vi "SP Convert 4.3 to 4.4.vi"(0 "S Parameter 4.3 Test Parameters":T2={"Stimulus"={"Use Instrument Settings"=FALSE, "Blank Frequencies"=FALSE, "Sweep Type"=enum."Linear", "Sweep"={"Fstart"=0.0, "Fstop"=0.0, "Units"=enum."Hz", "Points"=2}, "Power (dBm)"=999.0, "IFBW (Hz)"=-1.0, "Sweep Time (s)"=-1.0}, "Measurement"={"Auto Select"=FALSE, "Data Source"=enum."VNA", "Ports"=2, "Calibration"={"State"=FALSE, "String"=""}, "Parameters"=[]}, "De-Embed"={"De-Embed"=FALSE, "Adapters"=[]}, "Display"={"Lock Control"=FALSE, "Retain Settings"=FALSE, "Formatted Data"=FALSE, "Plot Orientation"=enum."Single", "Plot Controls"=[{"Trace Orientation"=enum."Overlay", "Frequency"={"Change Frequency"=FALSE, "Start"=500.0, "Stop"=1500.0, "Units"=enum."MHz"}, "Markers (MHz)"=[], "Traces"=[{"Trace On"=TRUE, "Measure"=0, "Format"=0, "Autoscale"=TRUE, "Reference"=0.0, "\nRefUnit"="dB/Div", "Position"=5.0, "Scale"=10.0, "ScaleUnit"="dB/Div", "LimitOn"=TRUE, "LimitFill"=FALSE, "Display Data"=0, "Show Markers"=FALSE, "SXX"=""}, {"Trace On"=TRUE, "Measure"=0, "Format"=0, "Autoscale"=TRUE, "Reference"=0.0, "\nRefUnit"="dB/Div", "Position"=5.0, "Scale"=10.0, "ScaleUnit"="dB/Div", "LimitOn"=TRUE, "LimitFill"=FALSE, "Display Data"=0, "Show Markers"=FALSE, "SXX"=""}]}, {"Trace Orientation"=enum."Overlay", "Frequency"={"Change Frequency"=FALSE, "Start"=500.0, "Stop"=1500.0, "Units"=enum."MHz"}, "Markers (MHz)"=[], "Traces"=[{"Trace On"=TRUE, "Measure"=0, "Format"=0, "Autoscale"=TRUE, "Reference"=0.0, "\nRefUnit"="dB/Div", "Position"=5.0, "Scale"=10.0, "ScaleUnit"="dB/Div", "LimitOn"=TRUE, "LimitFill"=FALSE, "Display Data"=0, "Show Markers"=FALSE, "SXX"=""}, {"Trace On"=TRUE, "Measure"=0, "Format"=0, "Autoscale"=TRUE, "Reference"=0.0, "\nRefUnit"="dB/Div", "Position"=5.0, "Scale"=10.0, "ScaleUnit"="dB/Div", "LimitOn"=TRUE, "LimitFill"=FALSE, "Display Data"=0, "Show Markers"=FALSE, "SXX"=""}]}, {"Trace Orientation"=enum."Overlay", "Frequency"={"Change Frequency"=FALSE, "Start"=500.0, "Stop"=1500.0, "Units"=enum."MHz"}, "Markers (MHz)"=[], "Traces"=[{"Trace On"=TRUE, "Measure"=0, "Format"=0, "Autoscale"=TRUE, "Reference"=0.0, "\nRefUnit"="dB/Div", "Position"=5.0, "Scale"=10.0, "ScaleUnit"="dB/Div", "LimitOn"=TRUE, "LimitFill"=FALSE, "Display Data"=0, "Show Markers"=FALSE, "SXX"=""}, {"Trace On"=TRUE, "Measure"=0, "Format"=0, "Autoscale"=TRUE, "Reference"=0.0, "\nRefUnit"="dB/Div", "Position"=5.0, "Scale"=10.0, "ScaleUnit"="dB/Div", "LimitOn"=TRUE, "LimitFill"=FALSE, "Display Data"=0, "Show Markers"=FALSE, "SXX"=""}]}, {"Trace Orientation"=enum."Overlay", "Frequency"={"Change Frequency"=FALSE, "Start"=500.0, "Stop"=1500.0, "Units"=enum."MHz"}, "Markers (MHz)"=[], "Traces"=[{"Trace On"=TRUE, "Measure"=0, "Format"=0, "Autoscale"=TRUE, "Reference"=0.0, "\nRefUnit"="dB/Div", "Position"=5.0, "Scale"=10.0, "ScaleUnit"="dB/Div", "LimitOn"=TRUE, "LimitFill"=FALSE, "Display Data"=0, "Show Markers"=FALSE, "SXX"=""}, {"Trace On"=TRUE, "Measure"=0, "Format"=0, "Autoscale"=TRUE, "Reference"=0.0, "\nRefUnit"="dB/Div", "Position"=5.0, "Scale"=10.0, "ScaleUnit"="dB/Div", "LimitOn"=TRUE, "LimitFill"=FALSE, "Display Data"=0, "Show Markers"=FALSE, "SXX"=""}]}]}, "Limits"=[]} {"Measurement"."Parameters"."Channel" min=0 max=32 step=1; "Stimulus"."Sweep Time (s)" format="%.3g"; "Display"."Plot Controls"."Traces"."Reference" format="%#.2g"; "Display"."Plot Controls"."Traces"."Display Data" items=["Data", "Memory", "Data/Memory"]; "Display"."Plot Controls"."Traces"."Format" items=["Log Mag", "Phase", "Delay", "Smith", "Polar", "Lin Mag", "SWR", "Loss", "Real", "Imaginary"]; "Display"."Plot Controls"."Traces"."Scale" min=0.001 step=1.0 format="%#.2g"; "Display"."Plot Controls"."Traces"."Position" min=0.0 max=10.0; "Display"."Plot Controls"."Frequency"."Stop" format="%.3g"; "Display"."Plot Controls"."Frequency"."Start" format="%.3g"}) -> (2 "S Parameter 4.4 - 4.5 Test Parameters":T1={"Stimulus"={"Use Instrument Settings"=FALSE, "Blank Frequencies"=FALSE, "Sweep Type"=enum."Linear", "Sweep"={"Fstart"=0.0, "Fstop"=0.0, "Units"=enum."Hz", "Points"=2}, "Power (dBm)"=999.0, "IFBW (Hz)"=-1.0, "Sweep Time (s)"=-1.0}, "Measurement"={"Auto Select"=TRUE, "Data Source"=enum."VNA", "Ports"=2, "Calibration"={"State"=FALSE, "String"=""}, "Parameters"=[]}, "De-Embed"={"De-Embed"=FALSE, "Adapters"=[]}, "Display"={"Lock Control"=FALSE, "Retain Settings"=TRUE, "Formatted Data"=FALSE, "Plot Orientation"=enum."Single", "Plot Controls"=[{"Trace Orientation"=enum."Overlay", "Frequency"={"Change Frequency"=FALSE, "Start"=500.0, "Stop"=1500.0, "Units"=enum."MHz"}, "Markers (MHz)"=[], "Traces"=[{"Trace On"=TRUE, "Measure"=0, "Format"=0, "Autoscale"=TRUE, "Reference"=0.0, "\nRefUnit"="dB/Div", "Position"=5.0, "Scale"=10.0, "ScaleUnit"="dB/Div", "LimitOn"=TRUE, "LimitFill"=FALSE, "Display Data"=0, "Show Markers"=FALSE, "SXX"=""}, {"Trace On"=TRUE, "Measure"=0, "Format"=0, "Autoscale"=TRUE, "Reference"=0.0, "\nRefUnit"="dB/Div", "Position"=5.0, "Scale"=10.0, "ScaleUnit"="dB/Div", "LimitOn"=TRUE, "LimitFill"=FALSE, "Display Data"=0, "Show Markers"=FALSE, "SXX"=""}]}, {"Trace Orientation"=enum."Overlay", "Frequency"={"Change Frequency"=FALSE, "Start"=500.0, "Stop"=1500.0, "Units"=enum."MHz"}, "Markers (MHz)"=[], "Traces"=[{"Trace On"=TRUE, "Measure"=0, "Format"=0, "Autoscale"=TRUE, "Reference"=0.0, "\nRefUnit"="dB/Div", "Position"=5.0, "Scale"=10.0, "ScaleUnit"="dB/Div", "LimitOn"=TRUE, "LimitFill"=FALSE, "Display Data"=0, "Show Markers"=FALSE, "SXX"=""}, {"Trace On"=TRUE, "Measure"=0, "Format"=0, "Autoscale"=TRUE, "Reference"=0.0, "\nRefUnit"="dB/Div", "Position"=5.0, "Scale"=10.0, "ScaleUnit"="dB/Div", "LimitOn"=TRUE, "LimitFill"=FALSE, "Display Data"=0, "Show Markers"=FALSE, "SXX"=""}]}, {"Trace Orientation"=enum."Overlay", "Frequency"={"Change Frequency"=FALSE, "Start"=500.0, "Stop"=1500.0, "Units"=enum."MHz"}, "Markers (MHz)"=[], "Traces"=[{"Trace On"=TRUE, "Measure"=0, "Format"=0, "Autoscale"=TRUE, "Reference"=0.0, "\nRefUnit"="dB/Div", "Position"=5.0, "Scale"=10.0, "ScaleUnit"="dB/Div", "LimitOn"=TRUE, "LimitFill"=FALSE, "Display Data"=0, "Show Markers"=FALSE, "SXX"=""}, {"Trace On"=TRUE, "Measure"=0, "Format"=0, "Autoscale"=TRUE, "Reference"=0.0, "\nRefUnit"="dB/Div", "Position"=5.0, "Scale"=10.0, "ScaleUnit"="dB/Div", "LimitOn"=TRUE, "LimitFill"=FALSE, "Display Data"=0, "Show Markers"=FALSE, "SXX"=""}]}, {"Trace Orientation"=enum."Overlay", "Frequency"={"Change Frequency"=FALSE, "Start"=500.0, "Stop"=1500.0, "Units"=enum."MHz"}, "Markers (MHz)"=[], "Traces"=[{"Trace On"=TRUE, "Measure"=0, "Format"=0, "Autoscale"=TRUE, "Reference"=0.0, "\nRefUnit"="dB/Div", "Position"=5.0, "Scale"=10.0, "ScaleUnit"="dB/Div", "LimitOn"=TRUE, "LimitFill"=FALSE, "Display Data"=0, "Show Markers"=FALSE, "SXX"=""}, {"Trace On"=TRUE, "Measure"=0, "Format"=0, "Autoscale"=TRUE, "Reference"=0.0, "\nRefUnit"="dB/Div", "Position"=5.0, "Scale"=10.0, "ScaleUnit"="dB/Div", "LimitOn"=TRUE, "LimitFill"=FALSE, "Display Data"=0, "Show Markers"=FALSE, "SXX"=""}]}]}, "Limits"=[]} {"Measurement"."Parameters"."Channel" min=0 max=32 step=1; "Measurement"."Parameters"."Parameter"."Stimulus Port" min=1 step=1; "Measurement"."Parameters"."Parameter"."Response Port" min=1 step=1; "Limits"."Parameter"."Stimulus Port" min=1 step=1; "Limits"."Parameter"."Response Port" min=1 step=1; "Stimulus"."Sweep Time (s)" format="%.3g"; "Display"."Plot Controls"."Traces"."Reference" format="%#.2g"; "Display"."Plot Controls"."Traces"."Display Data" items=["Data", "Memory", "Data/Memory"]; "Display"."Plot Controls"."Traces"."Format" items=["Log Mag", "Phase", "Expanded Phase", "Delay", "Smith", "Polar", "Lin Mag", "SWR", "Loss", "Real", "Imaginary"]; "Display"."Plot Controls"."Traces"."Scale" min=0.001 step=1.0 format="%#.2g"; "Display"."Plot Controls"."Traces"."Position" min=0.0 max=10.0; "Display"."Plot Controls"."Frequency"."Stop" format="%.3g"; "Display"."Plot Controls"."Frequency"."Start" format="%.3g"})   [LabVIEW 2011]
uses:
  TypeDefs/SP Test Parameters v4.3.ctl
  TypeDefs/SP Test Parameters v4.4-4.5.ctl
panel:
  # "Div"
  # "Div"
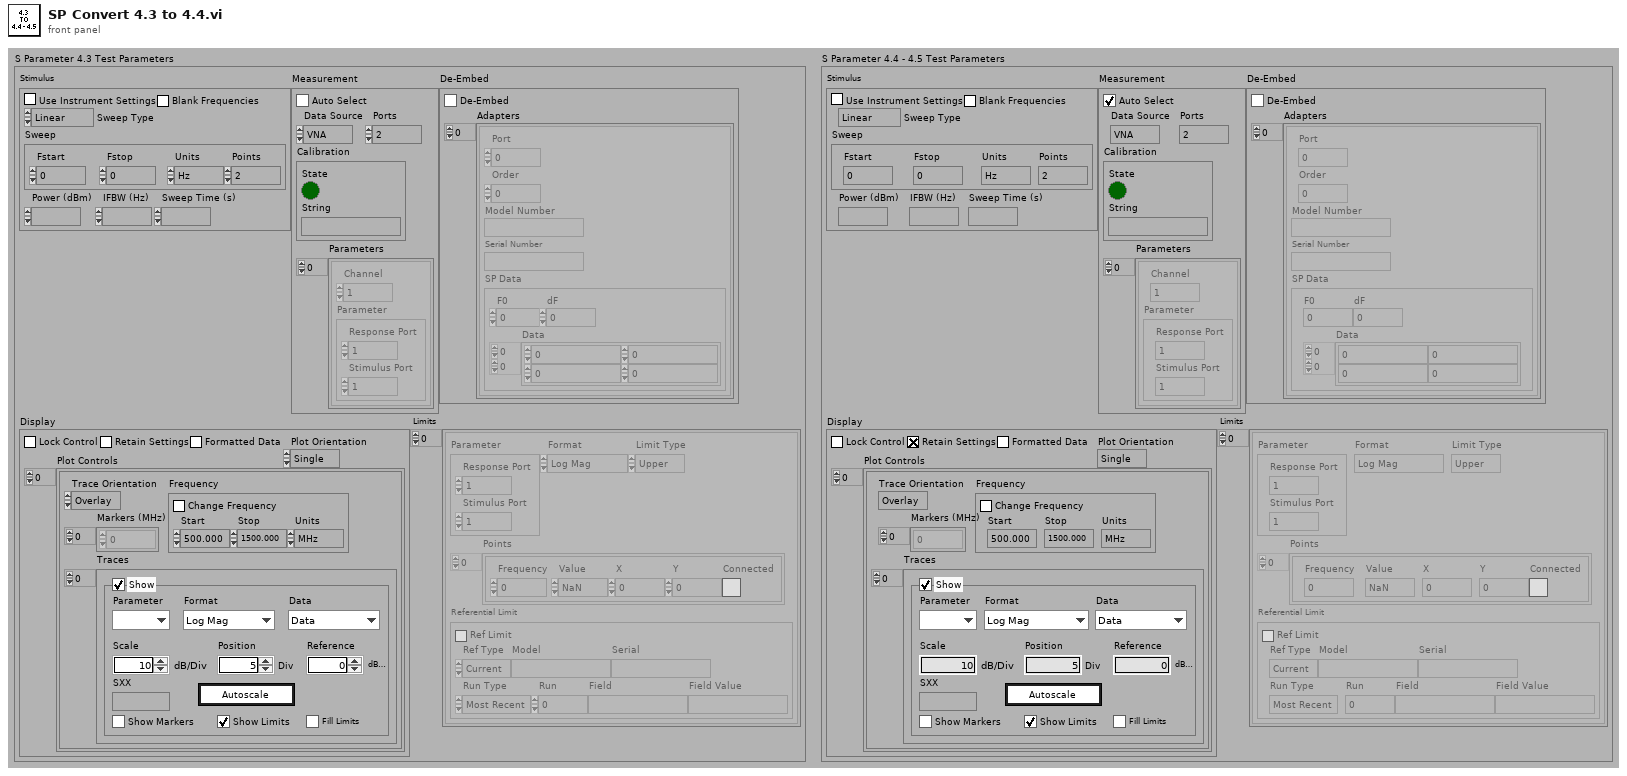
[diagram p1: front panel]
types:
  T1 = typedef "SP Test Parameters v4.4-4.5.ctl" = cluster{"Stimulus":cluster{"Use Instrument Settings":bool, "Blank Frequencies":bool, "Sweep Type":enum32{"Linear", "Logarithmic", "List", "Power", "CW"}, "Sweep":cluster{"Fstart":dbl, "Fstop":dbl, "Units":enum16{"Hz", "kHz", "MHz", "GHz", "Points"}, "Points":i32}, "Power (dBm)":dbl, "IFBW (Hz)":dbl, "Sweep Time (s)":dbl}, "Measurement":cluster{"Auto Select":bool, "Data Source":enum16{"VNA", "Data File"}, "Ports":i8, "Calibration":cluster{"State":bool, "String":string}, "Parameters":cluster{"Channel":i8, "Parameter":cluster{"Stimulus Port":i8, "Response Port":i8}}[]}, "De-Embed":cluster{"De-Embed":bool, "Adapters":cluster{"Port":i8, "Order":i8, "Model Number":string, "Serial Number":string, "SP Data":cluster{"F0":dbl, "dF":dbl, "Data":cdb[][]}}[]}, "Display":cluster{"Lock Control":bool, "Retain Settings":bool, "Formatted Data":bool, "Plot Orientation":enum32{"Single", "Dual", "Quad"}, "Plot Controls":cluster{"Trace Orientation":enum32{"Overlay", "Split"}, "Frequency":cluster{"Change Frequency":bool, "Start":dbl, "Stop":dbl, "Units":enum16{"Hz", "kHz", "MHz", "GHz", "Points"}}, "Markers (MHz)":dbl[], "Traces":cluster{"Trace On":bool, "Measure":i32, "Format":i32, "Autoscale":bool, "Reference":dbl, "\nRefUnit":string, "Position":dbl, "Scale":dbl, "ScaleUnit":string, "LimitOn":bool, "LimitFill":bool, "Display Data":u16, "Show Markers":bool, "SXX":string}[]}[]}, "Limits":cluster{"Parameter":cluster{"Stimulus Port":i8, "Response Port":i8}, "Format":enum16{"Log Mag", "Lin Mag", "SWR", "Phase", "Expanded Phase", "Delay", "Insertion Loss", "Isolation", "Return Loss"}, "Limit Type":enum16{"Upper", "Lower", "Delta"}, "Points":cluster{"Frequency":dbl, "Value":dbl, "X":dbl, "Y":dbl, "Connected":bool}[], "Referential Limit":cluster{"Ref Limit":bool, "Ref Type":enum16{"Current", "Specify"}, "Model":string, "Serial":string, "Run Type":enum16{"Most Recent", "Run #", "Match Field"}, "Run":i32, "Field":string, "Field Value":string}}[]}
  T2 = typedef "SP Test Parameters v4.3.ctl" = cluster{"Stimulus":cluster{"Use Instrument Settings":bool, "Blank Frequencies":bool, "Sweep Type":enum32{"Linear", "Logarithmic", "List", "Power", "CW"}, "Sweep":cluster{"Fstart":dbl, "Fstop":dbl, "Units":enum16{"Hz", "kHz", "MHz", "GHz"}, "Points":i32}, "Power (dBm)":dbl, "IFBW (Hz)":dbl, "Sweep Time (s)":dbl}, "Measurement":cluster{"Auto Select":bool, "Data Source":enum16{"VNA", "Data File"}, "Ports":i8, "Calibration":cluster{"State":bool, "String":string}, "Parameters":cluster{"Channel":i8, "Parameter":cluster{"Stimulus Port":i8, "Response Port":i8}}[]}, "De-Embed":cluster{"De-Embed":bool, "Adapters":cluster{"Port":i8, "Order":i8, "Model Number":string, "Serial Number":string, "SP Data":cluster{"F0":dbl, "dF":dbl, "Data":cdb[][]}}[]}, "Display":cluster{"Lock Control":bool, "Retain Settings":bool, "Formatted Data":bool, "Plot Orientation":enum32{"Single", "Dual", "Quad"}, "Plot Controls":cluster{"Trace Orientation":enum32{"Overlay", "Split"}, "Frequency":cluster{"Change Frequency":bool, "Start":dbl, "Stop":dbl, "Units":enum16{"Hz", "kHz", "MHz", "GHz"}}, "Markers (MHz)":dbl[], "Traces":cluster{"Trace On":bool, "Measure":i32, "Format":i32, "Autoscale":bool, "Reference":dbl, "\nRefUnit":string, "Position":dbl, "Scale":dbl, "ScaleUnit":string, "LimitOn":bool, "LimitFill":bool, "Display Data":u16, "Show Markers":bool, "SXX":string}[]}[]}, "Limits":cluster{"Parameter":cluster{"Stimulus Port":i8, "Response Port":i8}, "Format":enum16{"Log Mag", "Lin Mag", "SWR", "Phase", "Delay", "Insertion Loss", "Isolation", "Return Loss"}, "Limit Type":enum16{"Upper", "Lower", "Delta"}, "Points":cluster{"Frequency":dbl, "Value":dbl, "X":dbl, "Y":dbl, "Connected":bool}[], "Referential Limit":cluster{"Ref Limit":bool, "Ref Type":enum16{"Current", "Specify"}, "Model":string, "Serial":string, "Run Type":enum16{"Most Recent", "Run #", "Match Field"}, "Run":i32, "Field":string, "Field Value":string}}[]}
  T3 = cluster{"Trace Orientation":enum32{"Overlay", "Split"}, "Frequency":cluster{"Change Frequency":bool, "Start":dbl, "Stop":dbl, "Units":enum16{"Hz", "kHz", "MHz", "GHz", "Points"}}, "Markers (MHz)":dbl[], "Traces":cluster{"Trace On":bool, "Measure":i32, "Format":i32, "Autoscale":bool, "Reference":dbl, "\nRefUnit":string, "Position":dbl, "Scale":dbl, "ScaleUnit":string, "LimitOn":bool, "LimitFill":bool, "Display Data":u16, "Show Markers":bool, "SXX":string}[]}[]
  T4 = cluster{"Parameter":cluster{"Stimulus Port":i8, "Response Port":i8}, "Format":enum16{"Log Mag", "Lin Mag", "SWR", "Phase", "Expanded Phase", "Delay", "Insertion Loss", "Isolation", "Return Loss"}, "Limit Type":enum16{"Upper", "Lower", "Delta"}, "Points":cluster{"Frequency":dbl, "Value":dbl, "X":dbl, "Y":dbl, "Connected":bool}[], "Referential Limit":cluster{"Ref Limit":bool, "Ref Type":enum16{"Current", "Specify"}, "Model":string, "Serial":string, "Run Type":enum16{"Most Recent", "Run #", "Match Field"}, "Run":i32, "Field":string, "Field Value":string}}[]
  T5 = cluster{"Parameter":cluster{"Stimulus Port":i8, "Response Port":i8}, "Format":enum16{"Log Mag", "Lin Mag", "SWR", "Phase", "Expanded Phase", "Delay", "Insertion Loss", "Isolation", "Return Loss"}, "Limit Type":enum16{"Upper", "Lower", "Delta"}, "Points":cluster{"Frequency":dbl, "Value":dbl, "X":dbl, "Y":dbl, "Connected":bool}[], "Referential Limit":cluster{"Ref Limit":bool, "Ref Type":enum16{"Current", "Specify"}, "Model":string, "Serial":string, "Run Type":enum16{"Most Recent", "Run #", "Match Field"}, "Run":i32, "Field":string, "Field Value":string}}
  T6 = cluster{"Trace Orientation":enum32{"Overlay", "Split"}, "Frequency":cluster{"Change Frequency":bool, "Start":dbl, "Stop":dbl, "Units":enum16{"Hz", "kHz", "MHz", "GHz", "Points"}}, "Markers (MHz)":dbl[], "Traces":cluster{"Trace On":bool, "Measure":i32, "Format":i32, "Autoscale":bool, "Reference":dbl, "\nRefUnit":string, "Position":dbl, "Scale":dbl, "ScaleUnit":string, "LimitOn":bool, "LimitFill":bool, "Display Data":u16, "Show Markers":bool, "SXX":string}[]}
  T7 = cluster{"Trace On":bool, "Measure":i32, "Format":i32, "Autoscale":bool, "Reference":dbl, "\nRefUnit":string, "Position":dbl, "Scale":dbl, "ScaleUnit":string, "LimitOn":bool, "LimitFill":bool, "Display Data":u16, "Show Markers":bool, "SXX":string}[]
  T8 = cluster{"Use Instrument Settings":bool, "Blank Frequencies":bool, "Sweep Type":enum32{"Linear", "Logarithmic", "List", "Power", "CW"}, "Sweep":cluster{"Fstart":dbl, "Fstop":dbl, "Units":enum16{"Hz", "kHz", "MHz", "GHz"}, "Points":i32}, "Power (dBm)":dbl, "IFBW (Hz)":dbl, "Sweep Time (s)":dbl}
  T9 = cluster{"Auto Select":bool, "Data Source":enum16{"VNA", "Data File"}, "Ports":i8, "Calibration":cluster{"State":bool, "String":string}, "Parameters":cluster{"Channel":i8, "Parameter":cluster{"Stimulus Port":i8, "Response Port":i8}}[]}
  T10 = cluster{"De-Embed":bool, "Adapters":cluster{"Port":i8, "Order":i8, "Model Number":string, "Serial Number":string, "SP Data":cluster{"F0":dbl, "dF":dbl, "Data":cdb[][]}}[]}
  T11 = cluster{"Trace Orientation":enum32{"Overlay", "Split"}, "Frequency":cluster{"Change Frequency":bool, "Start":dbl, "Stop":dbl, "Units":enum16{"Hz", "kHz", "MHz", "GHz"}}, "Markers (MHz)":dbl[], "Traces":cluster{"Trace On":bool, "Measure":i32, "Format":i32, "Autoscale":bool, "Reference":dbl, "\nRefUnit":string, "Position":dbl, "Scale":dbl, "ScaleUnit":string, "LimitOn":bool, "LimitFill":bool, "Display Data":u16, "Show Markers":bool, "SXX":string}[]}[]
  T12 = cluster{"Parameter":cluster{"Stimulus Port":i8, "Response Port":i8}, "Format":enum16{"Log Mag", "Lin Mag", "SWR", "Phase", "Delay", "Insertion Loss", "Isolation", "Return Loss"}, "Limit Type":enum16{"Upper", "Lower", "Delta"}, "Points":cluster{"Frequency":dbl, "Value":dbl, "X":dbl, "Y":dbl, "Connected":bool}[], "Referential Limit":cluster{"Ref Limit":bool, "Ref Type":enum16{"Current", "Specify"}, "Model":string, "Serial":string, "Run Type":enum16{"Most Recent", "Run #", "Match Field"}, "Run":i32, "Field":string, "Field Value":string}}[]
  T13 = cluster{"Trace On":bool, "Measure":i32, "Format":i32, "Autoscale":bool, "Reference":dbl, "\nRefUnit":string, "Position":dbl, "Scale":dbl, "ScaleUnit":string, "LimitOn":bool, "LimitFill":bool, "Display Data":u16, "Show Markers":bool, "SXX":string}
  T14 = cluster{"Change Frequency":bool, "Start":dbl, "Stop":dbl, "Units":enum16{"Hz", "kHz", "MHz", "GHz"}}
  T15 = enum16{"Log Mag", "Lin Mag", "SWR", "Phase", "Delay", "Insertion Loss", "Isolation", "Return Loss"}
  T16 = cluster{"Frequency":dbl, "Value":dbl, "X":dbl, "Y":dbl, "Connected":bool}[]
  T17 = cluster{"Ref Limit":bool, "Ref Type":enum16{"Current", "Specify"}, "Model":string, "Serial":string, "Run Type":enum16{"Most Recent", "Run #", "Match Field"}, "Run":i32, "Field":string, "Field Value":string}
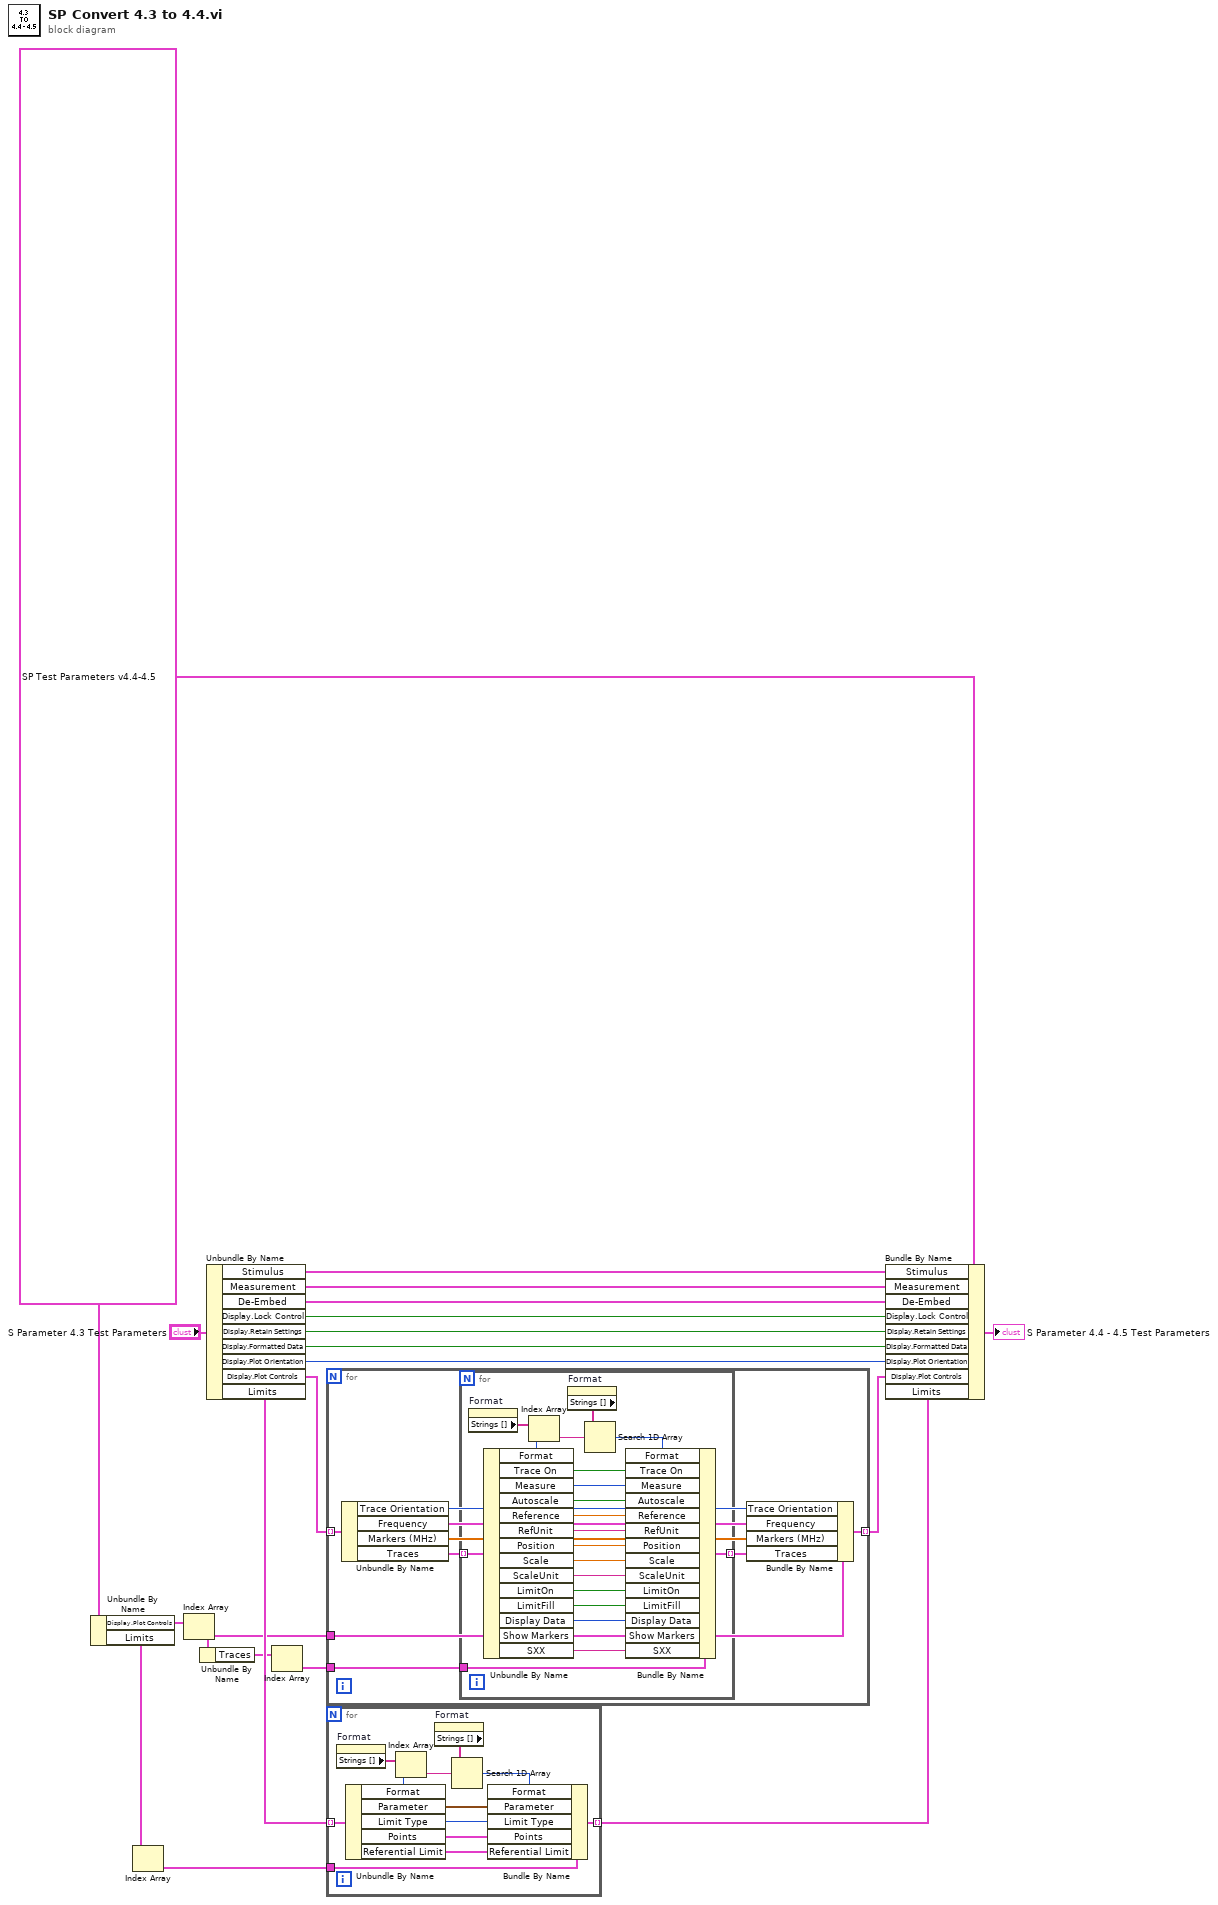
[diagram p0: block diagram]
diagram:
  w14 = T1 {"Stimulus"={"Use Instrument Settings"=FALSE, "Blank Frequencies"=FALSE, "Sweep Type"=enum."Linear", "Sweep"={"Fstart"=500.0, "Fstop"=1500.0, "Units"=enum."MHz", "Points"=2}, "Power (dBm)"=999.0, "IFBW (Hz)"=-1.0, "Sweep Time (s)"=-1.0}, "Measurement"={"Auto Select"=TRUE, "Data Source"=enum."VNA", "Ports"=2, "Calibration"={"State"=FALSE, "String"=""}, "Parameters"=[]}, "De-Embed"={"De-Embed"=FALSE, "Adapters"=[]}, "Display"={"Lock Control"=FALSE, "Retain Settings"=TRUE, "Formatted Data"=FALSE, "Plot Orientation"=enum."Single", "Plot Controls"=[{"Trace Orientation"=enum."Overlay", "Frequency"={"Change Frequency"=FALSE, "Start"=500.0, "Stop"=1500.0, "Units"=enum."MHz"}, "Markers (MHz)"=[], "Traces"=[{"Trace On"=TRUE, "Measure"=0, "Format"=0, "Autoscale"=TRUE, "Reference"=0.0, "\nRefUnit"="dB/Div", "Position"=5.0, "Scale"=10.0, "ScaleUnit"="dB/Div", "LimitOn"=TRUE, "LimitFill"=FALSE, "Display Data"=0, "Show Markers"=FALSE, "SXX"=""}, {"Trace On"=TRUE, "Measure"=0, "Format"=0, "Autoscale"=TRUE, "Reference"=0.0, "\nRefUnit"="dB/Div", "Position"=5.0, "Scale"=10.0, "ScaleUnit"="dB/Div", "LimitOn"=TRUE, "LimitFill"=FALSE, "Display Data"=0, "Show Markers"=FALSE, "SXX"=""}]}, {"Trace Orientation"=enum."Overlay", "Frequency"={"Change Frequency"=FALSE, "Start"=500.0, "Stop"=1500.0, "Units"=enum."MHz"}, "Markers (MHz)"=[], "Traces"=[{"Trace On"=TRUE, "Measure"=0, "Format"=0, "Autoscale"=TRUE, "Reference"=0.0, "\nRefUnit"="dB/Div", "Position"=5.0, "Scale"=10.0, "ScaleUnit"="dB/Div", "LimitOn"=TRUE, "LimitFill"=FALSE, "Display Data"=0, "Show Markers"=FALSE, "SXX"=""}, {"Trace On"=TRUE, "Measure"=0, "Format"=0, "Autoscale"=TRUE, "Reference"=0.0, "\nRefUnit"="dB/Div", "Position"=5.0, "Scale"=10.0, "ScaleUnit"="dB/Div", "LimitOn"=TRUE, "LimitFill"=FALSE, "Display Data"=0, "Show Markers"=FALSE, "SXX"=""}]}, {"Trace Orientation"=enum."Overlay", "Frequency"={"Change Frequency"=FALSE, "Start"=500.0, "Stop"=1500.0, "Units"=enum."MHz"}, "Markers (MHz)"=[], "Traces"=[{"Trace On"=TRUE, "Measure"=0, "Format"=0, "Autoscale"=TRUE, "Reference"=0.0, "\nRefUnit"="dB/Div", "Position"=5.0, "Scale"=10.0, "ScaleUnit"="dB/Div", "LimitOn"=TRUE, "LimitFill"=FALSE, "Display Data"=0, "Show Markers"=FALSE, "SXX"=""}, {"Trace On"=TRUE, "Measure"=0, "Format"=0, "Autoscale"=TRUE, "Reference"=0.0, "\nRefUnit"="dB/Div", "Position"=5.0, "Scale"=10.0, "ScaleUnit"="dB/Div", "LimitOn"=TRUE, "LimitFill"=FALSE, "Display Data"=0, "Show Markers"=FALSE, "SXX"=""}]}, {"Trace Orientation"=enum."Overlay", "Frequency"={"Change Frequency"=FALSE, "Start"=500.0, "Stop"=1500.0, "Units"=enum."MHz"}, "Markers (MHz)"=[], "Traces"=[{"Trace On"=TRUE, "Measure"=0, "Format"=0, "Autoscale"=TRUE, "Reference"=0.0, "\nRefUnit"="dB/Div", "Position"=5.0, "Scale"=10.0, "ScaleUnit"="dB/Div", "LimitOn"=TRUE, "LimitFill"=FALSE, "Display Data"=0, "Show Markers"=FALSE, "SXX"=""}, {"Trace On"=TRUE, "Measure"=0, "Format"=0, "Autoscale"=TRUE, "Reference"=0.0, "\nRefUnit"="dB/Div", "Position"=5.0, "Scale"=10.0, "ScaleUnit"="dB/Div", "LimitOn"=TRUE, "LimitFill"=FALSE, "Display Data"=0, "Show Markers"=FALSE, "SXX"=""}]}]}, "Limits"=[]} ("S Parameter Test Parameters")
  n1 = Unbundle By Name(w14) -> ("Display.Plot Controls"=w10:T3, "Limits"=w13:T4)
  n2 = Index Array(array=w13) -> (element=w12:T5)  [unwired: 1 in]
  n3 = Index Array(array=w10) -> (element=w7:T6)  [unwired: 1 in]
  n4 = Unbundle By Name(w7) -> ("Traces"=w9:T7)
  n5 = Unbundle By Name("S Parameter 4.3 Test Parameters") -> ("Stimulus"=w18:T8, "Measurement"=w17:T9, "De-Embed"=w16:T10, "Display.Lock Control"=w11:bool, "Display.Retain Settings"=w2:bool, "Display.Formatted Data"=w3:bool, "Display.Plot Orientation"=w4:enum32{"Single", "Dual", "Quad"}, "Display.Plot Controls"=w6:T11, "Limits"=w15:T12)
  n6 = Index Array(array=w9) -> (element=w8:T13)  [unwired: 1 in]
  n7 = for {
    tunnel: w6 -> [w29] mode=indexing
    tunnel: w8 -> [w27]
    tunnel: w7 -> [w26]
    tunnel: [w21] -> w5 mode=indexing
    n8 = Unbundle By Name(w29) -> ("Trace Orientation"=w25:enum32{"Overlay", "Split"}, "Frequency"=w24:T14, "Markers (MHz)"=w23:dbl[], "Traces"=w28:T7)
    n9 = for {
      tunnel: w28 -> [w50] mode=indexing
      tunnel: [w44] -> w22 mode=indexing
      tunnel: w27 -> [w43]
      n10 = property on="Format" class="Ring (strict)"() -> ("Strings []"=w49:string[])  [unwired: 2 in, 2 out]
      n11 = Unbundle By Name(w50) -> ("Format"=w48:i32, "Trace On"=w30:bool, "Measure"=w31:i32, "Autoscale"=w32:bool, "Reference"=w34:dbl, "RefUnit"=w33:string, "Position"=w35:dbl, "Scale"=w36:dbl, "ScaleUnit"=w37:string, "LimitOn"=w38:bool, "LimitFill"=w39:bool, "Display Data"=w40:u16, "Show Markers"=w41:bool, "SXX"=w42:string)
      n12 = Index Array(array=w49, index=w48) -> (element=w47:string)
      n13 = property on="Format" class="Ring (strict)"() -> ("Strings []"=w46:string[])  [unwired: 2 in, 2 out]
      n14 = Search 1D Array(1D array=w46, element=w47) -> (index of element=w45:i32)  [unwired: 1 out]
      n15 = Bundle By Name(cluster=w43, "Format"=w45, "Trace On"=w30, "Measure"=w31, "Autoscale"=w32, "Reference"=w34, "RefUnit"=w33, "Position"=w35, "Scale"=w36, "ScaleUnit"=w37, "LimitOn"=w38, "LimitFill"=w39, "Display Data"=w40, "Show Markers"=w41, "SXX"=w42) -> (w44:T13)
    }
    n16 = Bundle By Name(cluster=w26, "Trace Orientation"=w25, "Frequency"=w24, "Markers (MHz)"=w23, "Traces"=w22) -> (w21:T6)
  }
  n17 = for {
    tunnel: w15 -> [w62] mode=indexing
    tunnel: w12 -> [w57]
    tunnel: [w51] -> w1 mode=indexing
    n18 = property on="Format" class="Enum (strict)"() -> ("Strings []"=w61:string[])  [unwired: 2 in, 2 out]
    n19 = Unbundle By Name(w62) -> ("Format"=w60:T15, "Parameter"=w55:cluster{"Stimulus Port":i8, "Response Port":i8}, "Limit Type"=w56:enum16{"Upper", "Lower", "Delta"}, "Points"=w54:T16, "Referential Limit"=w53:T17)
    n20 = Index Array(array=w61, index=w60) -> (element=w59:string)
    n21 = property on="Format" class="Enum (strict)"() -> ("Strings []"=w58:string[])  [unwired: 2 in, 2 out]
    n22 = Search 1D Array(1D array=w58, element=w59) -> (index of element=w52:i32)  [unwired: 1 out]
    n23 = Bundle By Name(cluster=w57, "Format"=w52, "Parameter"=w55, "Limit Type"=w56, "Points"=w54, "Referential Limit"=w53) -> (w51:T5)
  }
  n24 = Bundle By Name(cluster=w14, "Stimulus"=w18, "Measurement"=w17, "De-Embed"=w16, "Display.Lock Control"=w11, "Display.Retain Settings"=w2, "Display.Formatted Data"=w3, "Display.Plot Orientation"=w4, "Display.Plot Controls"=w5, "Limits"=w1) -> (→"S Parameter 4.4 - 4.5 Test Parameters":T1)
